vi "On Data Message.vi"(8 "error in (no error)":errorcluster, 10 "Data Message":refnum<class "Data Message.lvclass">=refnum, 11 "This":refnum<class "Server.lvclass">) -> (0 "error out":errorcluster, 3 "This out":refnum<class "Server.lvclass">)   [LabVIEW 2023]
uses:
  Data Backplane/Data Message/Data Message.lvclass
  Server.lvclass
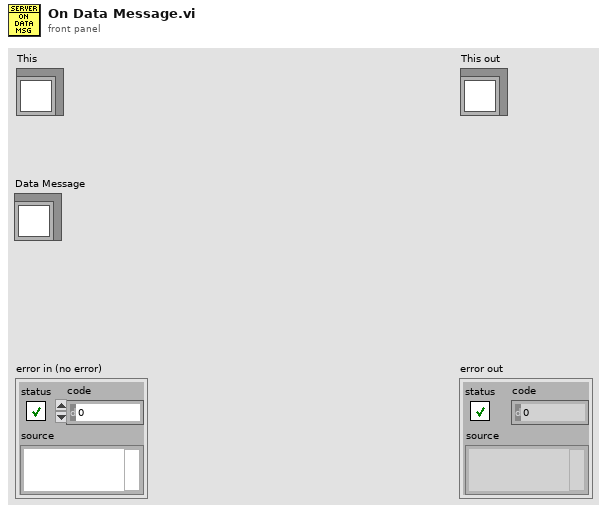
[diagram p1: front panel]
types:
  T1 = typedef "Server.lvclass/ObjectAttributes.ctl" = cluster{"Static Data":path, "MIME Types":variant, "Shutdown":bool, "API Queue":refnum<queue>, "ControlEndpoints":map{string, cluster{"Ref":refnum<vi>, "Mode":T2}}, "EventEndpoints":map{string, refnum<user-event>}}
  T2 = typedef "Server.lvclass/Control Ref Endpoint Access Mode.ctl" = enum16{"None", "Read/Write", "Read Only", "Write Only"}
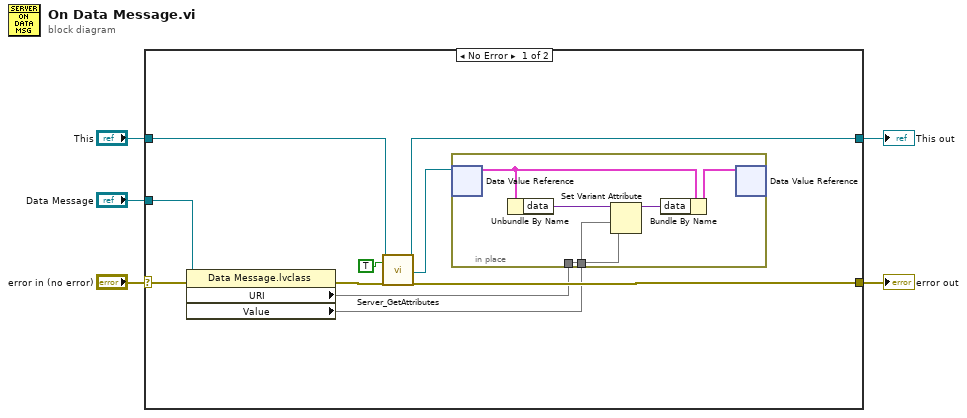
[diagram p0: block diagram]
diagram:
  n1 = case shown="No Error" "error in (no error)" {
    selector: "error in (no error)" -> [w14 w23]
    tunnel: [w11 w23] -> w4
    tunnel: [w10 w22] -> w2
    tunnel: "This" -> [w13 w22]
    tunnel: "Data Message" -> [w15 _]
    frame No Error {
      n2 = property class="Data Message.lvclass"(reference=w15, error in=w14) -> (error out=w12:errorcluster, "URI"=w7, "Value"=w6)  [unwired: 1 out]
      n3 = call "Server_GetAttributes.vi"("reference in"=w13, "OnlyGetDvrReference(False)"=TRUE, "error in (no error)"=w12) -> ("reference out"=w10:refnum<class "Server.lvclass">, "DataRef"=w8:refnum<data-value>, "error out"=w11:errorcluster)  [unwired: 13 in, 1 out]
      n4 = in-place {
        in-place-border: w7 -> [w20]
        in-place-border: w6 -> [w19]
        n5 = in-place-dvr #1(w8) -> (w18:T1)  [unwired: 1 out]
        n6 = Unbundle By Name(w18) -> ("data"=w21:variant)
        n7 = Set Variant Attribute(Variant=w21, name=w20, value=w19) -> (Variant out=w17:variant)  [unwired: 1 in, 2 out]
        n8 = Bundle By Name(cluster=w18, "data"=w17) -> (w16:T1)
        n9 = in-place-dvr #1(w16) -> ()  [unwired: 2 out]
      }
    }
    frame Error {
    }
  }
  "error out" <- w4
  "This out" <- w2
